vi "Pre-Process.vi"(8 "error in":errorcluster, 9 "Actual X Positions":dbl[](array[numeric]), 10 "New Data Points":T2, 11 "Scan Driver.lvclass in":refnum<class "Scan Driver.lvclass">) -> (0 "error out":errorcluster, 1 "Secondary Data":cluster{cluster{"x":T1, "x":T1}[]}[](array[cluster]), 2 "Primary Data":cluster{cluster{"x":T1, "x":T1}[]}[](array[cluster]), 3 "Scan Driver.lvclass out":refnum<class "Scan Driver.lvclass">)   [LabVIEW 2015, in "Scan Driver.lvclass"]
doc: "(Deprecated) Given a new data point, generate one or more auxilliary data points from a secondary source, e.g. a modulator Instrument or an internal computation algorithm. Return the updated onscreen scan graphs with the new data points."
uses:
  Scan Driver.lvclass
  Instruments/Utility Classes/Readable/Data Channels.ctl
  Instruments/Utility Classes/Readable/Data Channel.ctl
  Instruments/Utility Classes/Readable/Data Point.ctl
  Instruments/Utility Classes/Readable/Time.ctl
  Instruments/Utility Classes/Readable/X.ctl
  Scan Driver.lvclass/Scan Driver.ctl
  Scanners/Scanner/Scanner.lvclass
  Instruments/Utility Classes/Readable/Readable.lvclass
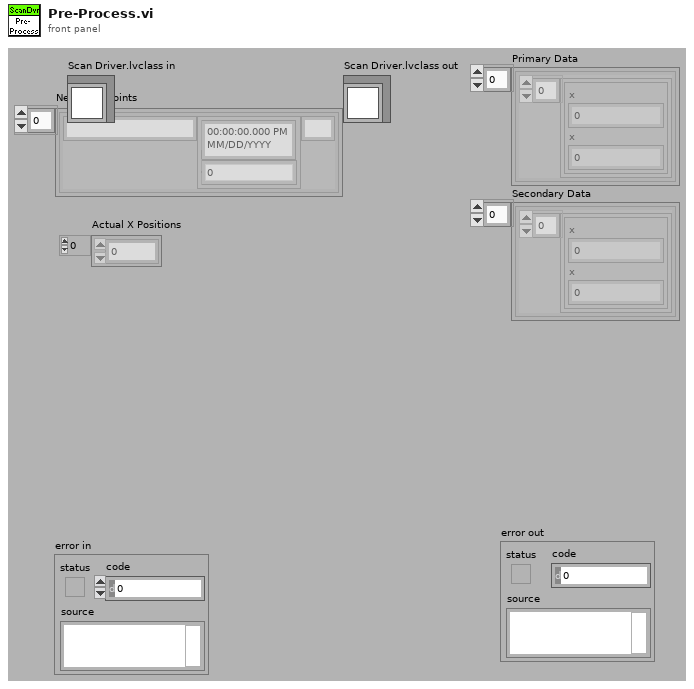
[diagram p1: front panel]
types:
  T1 = typedef "Readable.lvclass/X.ctl" = dbl
  T2 = typedef "Readable.lvclass/Data Channels.ctl" = T3[]
  T3 = typedef "Readable.lvclass/Data Channel.ctl" = cluster{"Name":string, "Data Point":T4, "Unit":string}
  T4 = typedef "Readable.lvclass/Data Point.ctl" = cluster{"t":T5, "x":T1}
  T5 = typedef "Readable.lvclass/Time.ctl" = timestamp
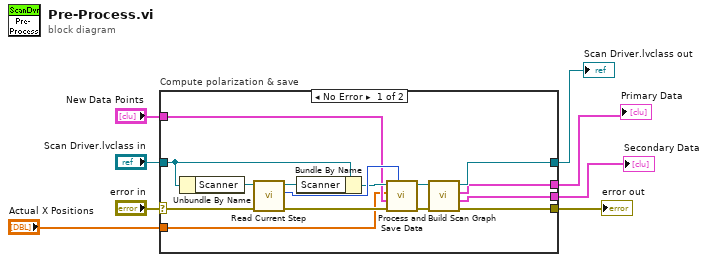
[diagram p0: block diagram]
diagram:
  n1 = case "Compute polarization & save" shown="No Error" "error in" {
    selector: "error in" -> [w12 w25]
    tunnel: "Actual X Positions" -> [w9 _]
    tunnel: "New Data Points" -> [w10 _]
    tunnel: [w22 _] -> w1
    tunnel: [w21 _] -> w2
    tunnel: [w18 w25] -> w6
    tunnel: [w23 w24] -> w4
    tunnel: "Scan Driver.lvclass in" -> [w17 w24]
    frame No Error {
      n2 = Unbundle By Name(w17) -> ("Scanner"=w16:refnum<class "Scanner.lvclass">)
      n3 = call-dynamic "Read Current Step.vi"("error in (no error)"=w12, "Scanner.lvclass in"=w16) -> ("error out"=w11:errorcluster, "Current Step"=w15:u32, "Scanner.lvclass out"=w13:refnum<class "Scanner.lvclass">)  [unwired: 7 out]
      n4 = Bundle By Name(cluster=w17, "Scanner"=w13) -> (w14:refnum<class "Scan Driver.lvclass">)
      n5 = call-dynamic "Process and Save Data.vi"("step#"=w15, "error in"=w11, "New Data Channels"=w10, "X-Vars"=w9, "Scan Driver.lvclass in"=w14) -> ("error out"=w19:errorcluster, "Scan Driver.lvclass out"=w20:refnum<class "Scan Driver.lvclass">)  [unwired: 3 in, 2 out]
      n6 = call-dynamic "Build Scan Graph.vi"("error in"=w19, "Scan Driver in"=w20) -> ("error out"=w18:errorcluster, "Secondary Data"=w21:cluster{cluster{"x":T1, "x":T1}[]}[], "Primary Data"=w22:cluster{cluster{"x":T1, "x":T1}[]}[], "Scan Driver out"=w23:refnum<class "Scan Driver.lvclass">)  [unwired: 4 in, 2 out]
    }
    frame Error {
    }
  }
  "Scan Driver.lvclass out" <- w4
  "error out" <- w6
  "Primary Data" <- w1
  "Secondary Data" <- w2
